vi "ProgramAnLEDToBlink.vi"   [LabVIEW 2012]
types:
  T1 = typedef "BotSpeak_Control.ctl" = cluster{"Address":string, "Reply EOF":string, "Hardware":string, "Retries":i8, "Timeout":i32}
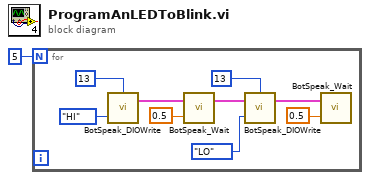
[diagram p0: block diagram]
diagram:
  n1 = for {
    N: 5 -> [_]
    n2 = call <userlib>:"BotSpeak_DIOWrite.vi"("State"=enum32{"LO", "HI"}."HI", "DIO Line"=u32 13) -> ("Bot Settings"=w7:T1)  [unwired: 1 in, 1 out]
    n3 = call <userlib>:"BotSpeak_Wait.vi"("Wait (sec)"=0.5, "Bot Settings"=w7) -> ("Bot Settings"=w6:T1)  [unwired: 1 in]
    n4 = call <userlib>:"BotSpeak_DIOWrite.vi"("State"=enum32{"LO", "HI"}."LO", "Bot Settings"=w6, "DIO Line"=u32 13) -> ("Bot Settings"=w3:T1)  [unwired: 1 out]
    n5 = call <userlib>:"BotSpeak_Wait.vi"("Wait (sec)"=0.5, "Bot Settings"=w3) -> ()  [unwired: 1 in, 1 out]
  }
